vi "Launch Process.vi"(8 "error in (no error)":errorcluster, 11 "LogEngine.lvclass":refnum<class "LogEngine.lvclass">) -> (0 "error out":errorcluster, 3 "LogEngine.lvclass":refnum<class "LogEngine.lvclass">)   [LabVIEW 2017, in "LogEngine.lvclass"]
doc: "Developed by Kevin Thompson\nkevin@thompsonengineering.net\n\nCopyright 2018-2020\nThompson Engineering, LLC"
uses:
  LogEngine.lvclass
  Process_LogEngine.vi
panel:
  out "timed out?":bool
  out "sync with process?":bool
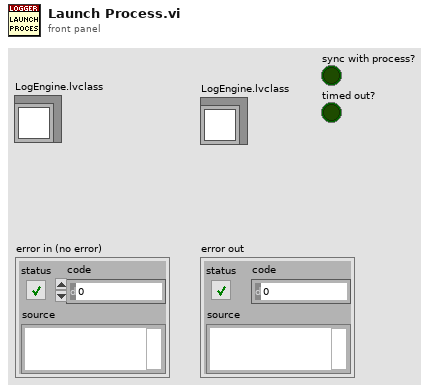
[diagram p1: front panel]
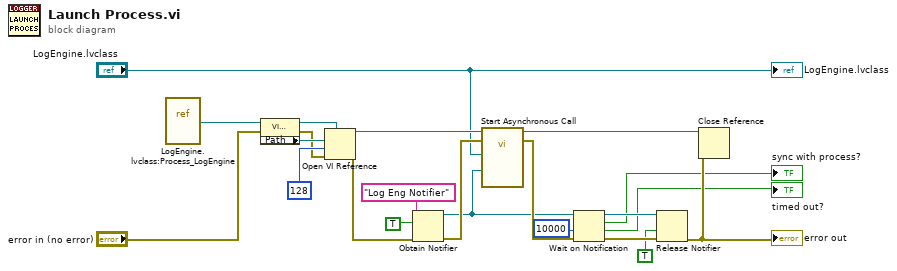
[diagram p0: block diagram]
diagram:
  n1 = vi-ref "LogEngine.lvclass:Process_LogEngine.vi"() -> (w20:refnum<vi>)
  n2 = property class="VI (strict)"(reference=w20, error in="error in (no error)") -> (reference out=w18:refnum<vi>, error out=w11:errorcluster, "Path"=w19:path)
  n3 = Open VI Reference(type specifier VI Refnum (for type only)=w18, vi path=w19, options=128, error in (no error)=w11) -> (vi reference=w16:refnum<vi>, error out=w12:errorcluster)  [unwired: 2 in]
  n4 = Obtain Notifier(name (unnamed)="Log Eng Notifier", notification data type=TRUE, error in (no error)=w12) -> (notifier out=w5:refnum<notifier>, error out=w14:errorcluster)  [unwired: 1 in, 1 out]
  n5 = call-by-ref "Start Asynchronous Call"(reference=w16, error in=w14, "start process sync notifier"=w5, "LogEngine.lvclass"="LogEngine.lvclass") -> (reference out=w7:refnum<vi>, error out=w13:errorcluster)  [unwired: 9 in, 1 out]
  n6 = Wait on Notification(notifier=w5, timeout in ms (-1)=10000, error in (no error)=w13) -> (notifier out=w8:refnum<notifier>, notification=→"sync with process?":bool, timed out?=→"timed out?":bool, error out=w9:errorcluster)  [unwired: 1 in]
  n7 = Release Notifier(notifier=w8, force destroy? (F)=TRUE, error in (no error)=w9) -> (error out=w22:errorcluster)  [unwired: 2 out]
  "error out" <- w22
  n8 = Close Reference(reference=w7, error in (no error)=w22) -> ()  [unwired: 1 out]
  "LogEngine.lvclass" <- "LogEngine.lvclass"
